vi "v_local.vi"() -> ()   [LabVIEW 2020]
panel:
  out "Temperatura":dbl[](array[numeric])
  in  "Thermometer":dbl(slide) scale=0.0..100.0
  out "String 2":string
  out "Led":bool
  in  "Pulsador":bool
  in  "stop":bool
  out "Numeric 3":i32
  out "Numeric 2":i32
  out "Numeric":i32
  # "Variables Locales en Labview"
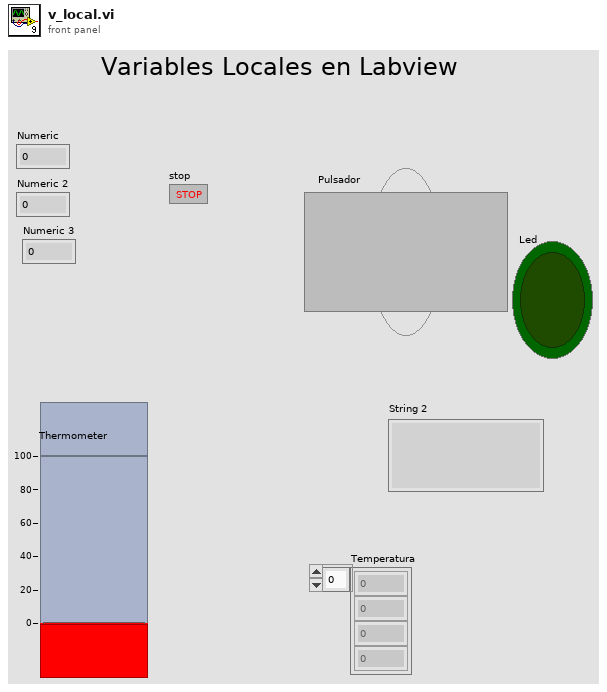
[diagram p1: front panel]
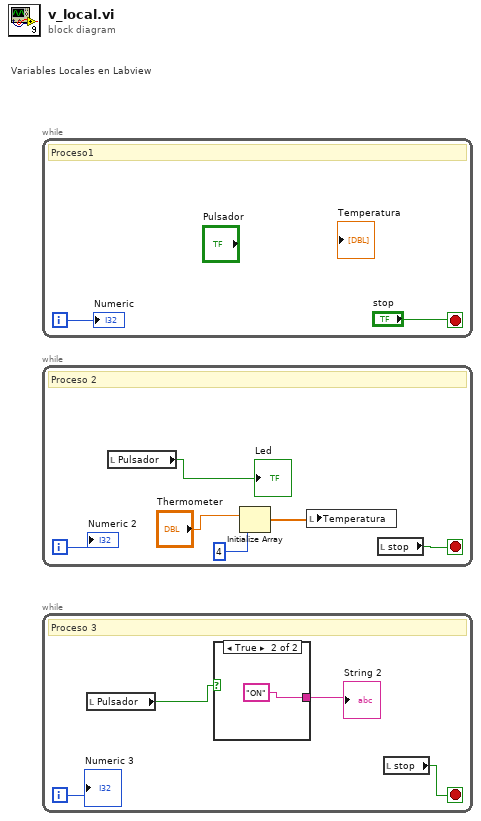
[diagram p0: block diagram]
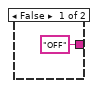
[diagram p2: hidden frame]
diagram:
  # "Variables Locales en Labview"
  n1 = while {
    i -> [w2]
    stop <- "stop" stop-if-true
    # "Proceso1"
    "Numeric" <- w2
  }
  n2 = while {
    i -> [w8]
    stop <- w7 stop-if-true
    # "Proceso 2"
    n3 = local read "Pulsador"() -> (→"Led":bool)
    n4 = Initialize Array("Thermometer", 4 ("dimension size")) -> (w3:dbl[])
    n5 = local write "Temperatura"(w3) -> ()
    n6 = local read "stop"() -> (w7:bool)
    "Numeric 2" <- w8
  }
  n7 = while {
    i -> [w12]
    stop <- w11 stop-if-true
    # "Proceso 3"
    n8 = local read "Pulsador"() -> (w10:bool)
    n9 = case shown="True" w10 {
      tunnel: ["OFF" "ON"] -> w9
      frame False {
      }
      frame True {
      }
    }
    "String 2" <- w9
    n10 = local read "stop"() -> (w11:bool)
    "Numeric 3" <- w12
  }
